vi "Read FIFOs.vi"(7 "Mode":T1, 8 "error in (no error)":errorcluster, 11 "RT Data in":T2 {"Label Transfer Config"."Block Data Refs"."Data Reference" format="%.0x"; "Status Config"."HWOut Dur Ref" format="%.0x"; "Status Config"."HWIn Dur Ref" format="%.0x"; "Status Config"."Error Data Ref" format="%.0x"; "HWOutput Channels"."Labels Settings"."Label" format="%.0o"; "HWInput Channels"."Labels Settings"."Label" format="%.0o"}) -> (0 "error out":errorcluster, 1 "Empty From HWOut":bool, 2 "Empty From HWIn":bool, 3 "RT Data out":T2 {"Label Transfer Config"."Block Data Refs"."Data Reference" format="%.0x"; "Status Config"."HWOut Dur Ref" format="%.0x"; "Status Config"."HWIn Dur Ref" format="%.0x"; "Status Config"."Error Data Ref" format="%.0x"; "HWOutput Channels"."Labels Settings"."Label" format="%.0o"; "HWInput Channels"."Labels Settings"."Label" format="%.0o"})   [LabVIEW 2012, in "AIT 429 Engine.lvlib"]
uses:
  AIT 429 Engine.lvlib
  RT Controls/RT Data.ctl
  RT Controls/RT HW Channel.ctl
  RT Controls/RT Label Settings.ctl
  Shared/Controls and Global/Label.ctl
  Shared/Controls and Global/transferPeriod.ctl
  RT Controls/Driver Data.ctl
  RT Controls/RT Word Settings.ctl
  <vilib>/NI Veristand/Custom Device API/Block Data Reference.ctl
  <vilib>/NI Veristand/Custom Device API/Data Reference.ctl
  RT Controls/RT Param Setting.ctl
  Shared/Controls and Global/Start Bit.ctl
  Shared/Controls and Global/Number of Bits.ctl
  Shared/Controls and Global/TransferType.ctl
  RT Controls/Error Qs.ctl
  RT Controls/Status Channels Config.ctl
  RT Controls/FIFO.ctl
  RT Controls/Label Transfer Config.ctl
  SEA 9811 FPGA driver/RT/Typdefs/SEA9811_RT_data_cluster.ctl
  SEA 9811 FPGA driver/RT/Typdefs/FPGA ref.ctl
  SEA 9811 FPGA driver/RT/Typdefs/channel.ctl
  SEA 9811 FPGA driver/RT/Typdefs/received word.ctl
  RT Controls/ReadWrite Selector.ctl
  Shared/ARINC 429 Shared.lvlib
  <vilib>/NI Veristand/Custom Device API/Custom Device API.lvlib
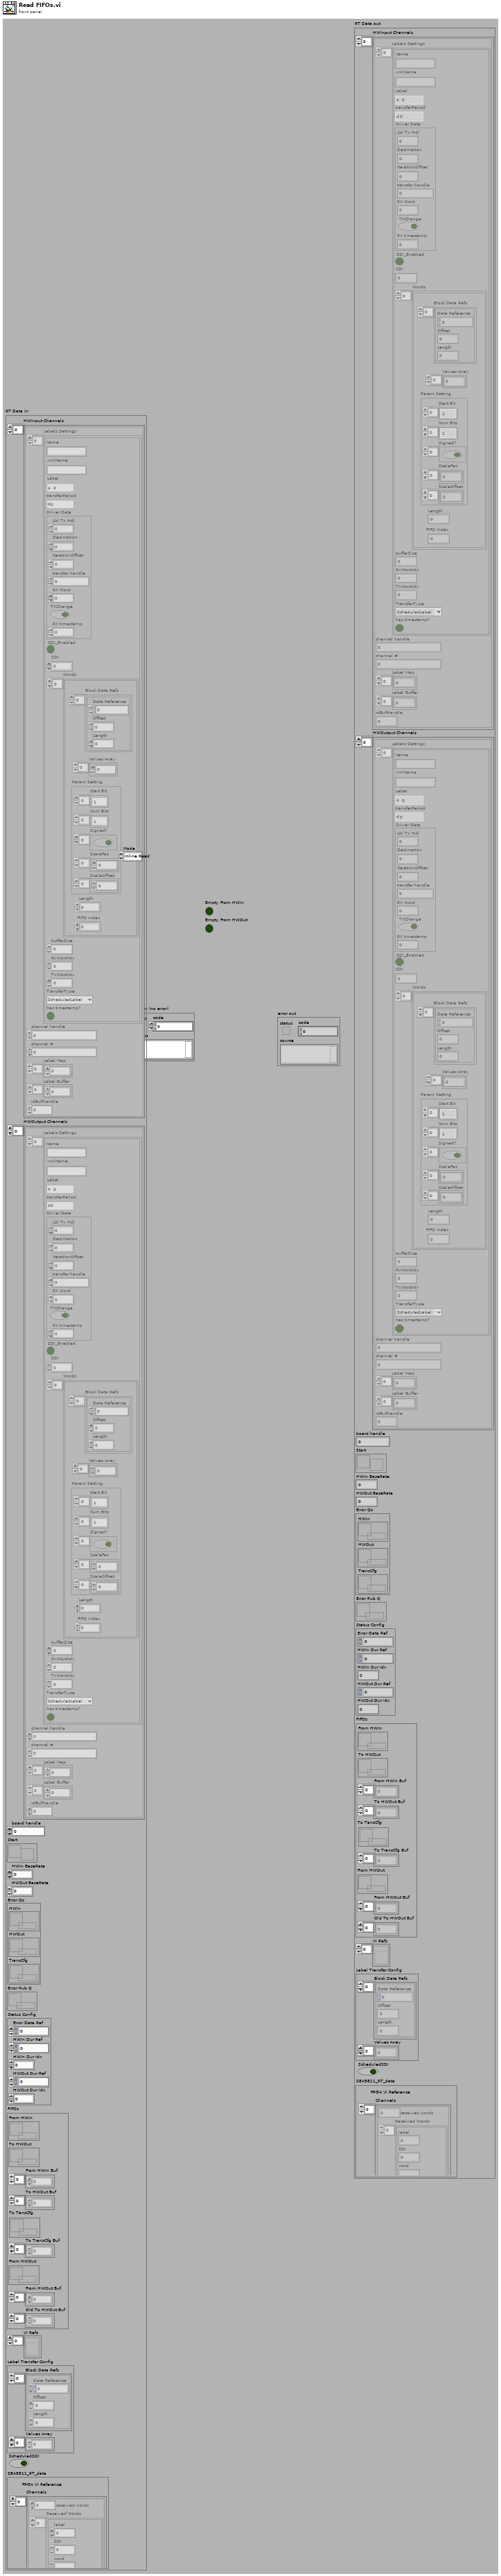
[diagram p1: front panel]
types:
  T1 = typedef "AIT 429 Engine.lvlib/ReadWrite Selector.ctl" = enum16{"Inline Read", "Inline Write", "Async HWIn", "Async HWOut"}
  T2 = typedef "AIT 429 Engine.lvlib/RT Data.ctl" = cluster{"HWInput Channels":T3[], "HWOutput Channels":T3[], "board handle":u32, "Start":refnum<notifier>, "HWIn BaseRate":i64, "HWOut BaseRate":i64, "Error Qs":T15, "Error Pub Q":refnum<queue>, "Status Config":T16, "FIFOs":T17, "VI Refs":refnum<vi>[], "Label Transfer Config":T18, "ScheduledSDI":bool, "SEA9811_RT_data":T19}
  T3 = typedef "AIT 429 Engine.lvlib/RT HW Channel.ctl" = cluster{"Labels Settings":T4[], "channel handle":u32, "channel #":u16, "Label Map":i32[], "Label Buffer":u32[], "rdBufHandle":u32}
  T4 = typedef "AIT 429 Engine.lvlib/RT Label Settings.ctl" = cluster{"Name":string, "xmlName":string, "Label":T5, "transferPeriod":T6, "Driver Data":T7, "SDI_Enabled":bool, "SDI":u8, "Words":T8[], "bufferSize":u32, "RxWordIdx":i32, "TxWordIdx":i32, "TransferType":T14, "has timestamp?":bool}
  T5 = typedef "ARINC 429 Shared.lvlib/Label.ctl" = u8
  T6 = typedef "ARINC 429 Shared.lvlib/transferPeriod.ctl" = u32
  T7 = typedef "AIT 429 Engine.lvlib/Driver Data.ctl" = cluster{"Lbl Tx Hdl":u32, "Decimation":i32, "IterationOffset":i32, "transfer handle":u32, "RX Word":u32, "TXChange":bool, "RX timestamp":dbl}
  T8 = typedef "AIT 429 Engine.lvlib/RT Word Settings.ctl" = cluster{"Block Data Refs":T9[], "Values Array":dbl[], "Length":i32, "FIFO Index":i32, "Param Setting":T11}
  T9 = typedef "Custom Device API.lvlib/Block Data Reference.ctl" = cluster{"Data Reference":T10, "Offset":i32, "Length":i32}
  T10 = typedef "Custom Device API.lvlib/Data Reference.ctl" = i32
  T11 = typedef "AIT 429 Engine.lvlib/RT Param Setting.ctl" = cluster{"Start Bit":T12[], "Num Bits":T13[], "Signed?":bool[], "ScaleFac":dbl[], "ScaleOffset":dbl[]}
  T12 = typedef "ARINC 429 Shared.lvlib/Start Bit.ctl" = i32
  T13 = typedef "ARINC 429 Shared.lvlib/Number of Bits.ctl" = i32
  T14 = typedef "ARINC 429 Shared.lvlib/TransferType.ctl" = enum16{"ScheduledLabel", "Acyclic", "Block", "Strobe"}
  T15 = typedef "AIT 429 Engine.lvlib/Error Qs.ctl" = cluster{"HWIn":refnum<queue>, "HWOut":refnum<queue>, "TransCfg":refnum<queue>}
  T16 = typedef "AIT 429 Engine.lvlib/Status Channels Config.ctl" = cluster{"Error Data Ref":T10, "HWIn Dur Ref":T10, "HWIn Dur Idx":i32, "HWOut Dur Ref":T10, "HWOut Dur Idx":i32}
  T17 = typedef "AIT 429 Engine.lvlib/FIFO.ctl" = cluster{"From HWIn":refnum<k33>, "To HWOut":refnum<k33>, "From HWIn Buf":dbl[], "To HWOut Buf":dbl[], "To TansCfg":refnum<k33>, "To TransCfg Buf":dbl[], "From HWOut":refnum<k33>, "From HWOut Buf":dbl[], "Old To HWOut Buf":dbl[]}
  T18 = typedef "AIT 429 Engine.lvlib/Label Transfer Config.ctl" = cluster{"Block Data Refs":T9[], "Values Array":dbl[]}
  T19 = typedef "SEA9811_RT_data_cluster.ctl" = cluster{"FPGA VI Reference":T20, "Channels":T21[]}
  T20 = typedef "FPGA ref.ctl" = refnum<k20>
  T21 = typedef "channel.ctl" = cluster{"received words":u32, "Received Words":T22[]}
  T22 = typedef "received word.ctl" = cluster{"label":u8, "SDI":u8, "word":u32, "timestamp":dbl}
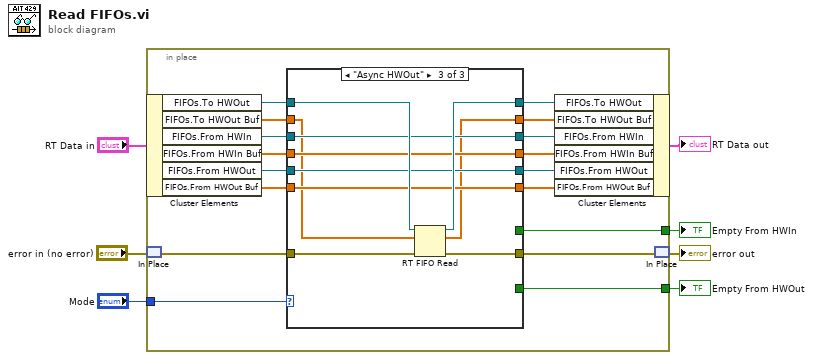
[diagram p0: block diagram]
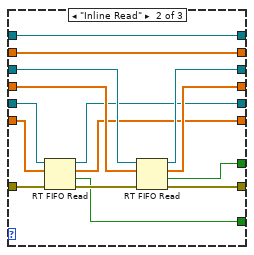
[diagram p3: hidden frame]
diagram:
  n1 = in-place {
    in-place-border: "Mode" -> [w18]
    in-place-border: [w9] -> w2
    in-place-border: [w8] -> w1
    n2 = in-place-cluster #1("RT Data in") -> ("FIFOs.To HWOut"=w17:refnum<k33>, "FIFOs.To HWOut Buf"=w16:dbl[], "FIFOs.From HWIn"=w24:refnum<k33>, "FIFOs.From HWIn Buf"=w23:dbl[], "FIFOs.From HWOut"=w13:refnum<k33>, "FIFOs.From HWOut Buf"=w12:dbl[])
    n3 = in-place-match #2("error in (no error)") -> (w20:errorcluster)
    n4 = case shown="\"Async HWOut\"" w18 {
      tunnel: w24 -> [w30 w46 w52]
      tunnel: w23 -> [w31 w45 w53]
      tunnel: [w31 w44 w53] -> w22
      tunnel: [w30 w43 w52] -> w21
      tunnel: w20 -> [w29 w42 w49]
      tunnel: [w29 w41 w56] -> w19
      tunnel: w17 -> [w27 w40 w55]
      tunnel: w16 -> [w28 w39 w48]
      tunnel: [w27 w40 w54] -> w15
      tunnel: [w28 w39 w47] -> w14
      tunnel: w13 -> [w26 w37 w51]
      tunnel: w12 -> [w25 w36 w50]
      tunnel: [w26 w35 w51] -> w11
      tunnel: [w25 w34 w50] -> w10
      tunnel: [_ w33 _] -> w9
      tunnel: [_ w32 _] -> w8
      frame Default {
      }
      frame "Inline Read" {
        n5 = RT FIFO Read(0:w37, 1:w36, 3:w42) -> (8:w35:refnum<k33>, 9:w34:dbl[], 10:w32:bool, 11:w38:errorcluster)  [unwired: 1 in, 1 out]
        n6 = RT FIFO Read(0:w46, 1:w45, 3:w38) -> (8:w43:refnum<k33>, 9:w44:dbl[], 10:w33:bool, 11:w41:errorcluster)  [unwired: 1 in, 1 out]
      }
      frame "Async HWOut" {
        n7 = RT FIFO Read(0:w55, 1:w48, 3:w49) -> (8:w54:refnum<k33>, 9:w47:dbl[], 11:w56:errorcluster)  [unwired: 1 in, 2 out]
      }
    }
    n8 = in-place-cluster #1("FIFOs.To HWOut"=w15, "FIFOs.To HWOut Buf"=w14, "FIFOs.From HWIn"=w21, "FIFOs.From HWIn Buf"=w22, "FIFOs.From HWOut"=w11, "FIFOs.From HWOut Buf"=w10) -> (→"RT Data out":T2)
    n9 = in-place-match #2(w19) -> (→"error out":errorcluster)
  }
  "Empty From HWIn" <- w2
  "Empty From HWOut" <- w1
